vi "Window.vi"() -> ()   [LabVIEW 2010]
uses:
  <vilib>/Platform/TimedLoop/XDataNode/XDataNode.xnode
  <vilib>/Platform/TimedLoop/XDataNode/timing_clust.ctl
  <vilib>/Platform/TimedLoop/XDataNode/nitl_modes.ctl
  <vilib>/Platform/TimedLoop/XDataNode/wakeup.ctl
  LabView Dec.8/LabView Dec.8/SubVi's/Time Variable.vi
  SubVi's/Time Zone Offset.vi
  <vilib>/Utility/file.llb/Write To Spreadsheet File (string).vi
  LabView Dec.8/LabView Dec.8/SubVi's/Plot Variable.vi
  <vilib>/Platform/TimedLoop/XDataNode/XDNodeRunTimeDep.lvlib
  <vilib>/gmath/NI_Gmath.lvlib
  <vilib>/Analysis/NI_AALPro.lvlib
  LabView Dec.8/LabView Dec.8/SQL project lib.lvlib
  <vilib>/addons/database/NI_Database_API.lvlib
panel:
  in  "Background":bool
  in  "Grab Since Start":bool
  in  "Start Time":timestamp format="%<%H:%M:%S\n%x>T"
  in  "End Time":timestamp format="%<%H:%M:%S\n%x>T"
  in  "Grab Interval":bool
  in  "Fit":bool
  in  "Log(Y)":bool
  in  "Log(X)":bool
  in  "Remove":bool[](array[boolean])
  in  "Scatter/Histogram":bool=TRUE
  in  "bins":i32=250
  in  "min":dbl format="%_3g"
  in  "max":dbl=10.0 format="%0.2f"
  out "Current Data":dbl[](array[numeric])
  in  "Plot Scale":string[](array[string])=["y", "y", "y", "y", "y", "y", "y", "y", "y", "y", "y", "y", "y", "y", "y", "y", "y", "y", "y", "y", "y", "y", "y", "y", "y", "y", "y", "y", "y", "y", "y", "y", "y", "y", "y", "y", "y", "y", "y", "y", "y", "y", "y", "y", "y", "y", "y", "y", "y", "y", "y", "y", "y", "y", "y", "y", "y", "y", "y", "y", "y", "y", "y", "y", "y", "y", "y", "y", "y", "y", "y", "y", "y", "y", "y", "y", "y", "y", "y", "y", "y", "y", "y", "y", "y", "y", "y", "y", "y", "y", "y", "y", "y", "y", "y", "y", "y", "y", "y", "y", "y"]
  in  "Clear":bool
  out "Data Channel Name":string[](array[string])
  out "Realtime?":bool
  in  "Autoscale All":bool
  in  "output cluster":T1
  in  "Show Comments":bool
  in  "VI Refnum":refnum<vi>
  in  "Select Path (dialog if empty) 2":path
  in  "Save Front Panel Image":bool
  in  "Select Path (dialog if empty)":path
  in  "Write Data to \nLocal File":bool
  in  "Points to Plot":i32=4000
  in  "Realtime?":bool
  in  "Sent Array":cluster{dbl[], dbl[]}[](graph)
  in  "New String":string[](array[string])
  out "Plot":cluster{dbl[], dbl[]}[](graph)
  in  "New Data?":dbl=0.1
  out "Scaled Plot":cluster{dbl[], dbl[]}[](graph)
  # "Hist. Controls:"
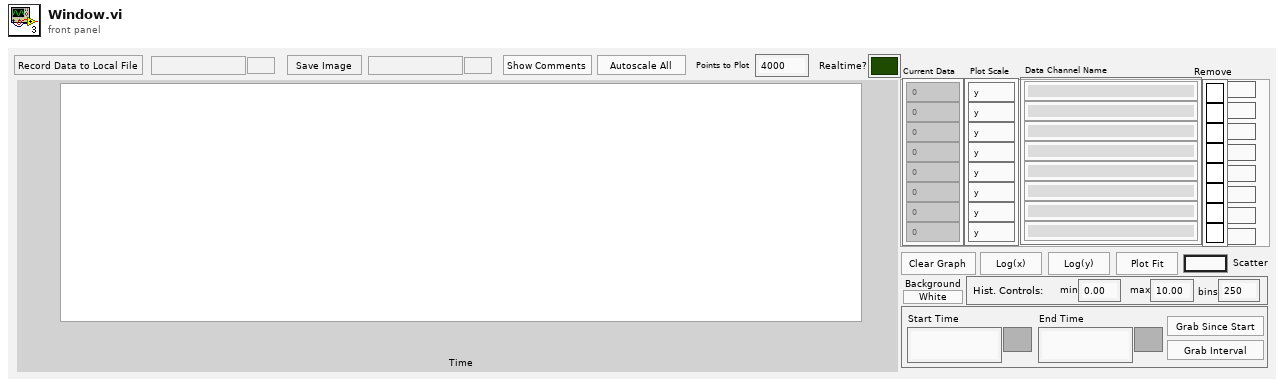
[diagram p1: front panel]
types:
  T1 = cluster{"Name":string, "Color":u32, "Style":u8, "Point Style":u8, "Name Visible":bool, "Allow Drag":bool, "Annotation Mode":u32, "Plot":i32, "Index":i32, "Position":cluster{"X":dbl, "Y":dbl}, "X Scale":u32, "Y Scale":u32, "Show Arrow":bool, "Lock Name":bool, "Plot Area":i32, "Label Offset":cluster{"X":dbl, "Y":dbl}}
  T2 = typedef "XDNodeRunTimeDep.lvlib/timing_clust.ctl" = cluster{"Expected End [f-1]":u64, "Actual End [f-1]":u64, "Finished Late? [f-1]":bool, "Expected End [i-1]":u64, "Actual End [i-1]":u64, "Finished Late? [i-1]":bool, "Expected Start [i]":u64, "Actual Start [i]":u64, "Expected Start [f]":u64, "Actual Start [f]":u64, "Source Name":string, "Structure Name":string, "Period":i64, "Deadline":i64, "Offset":i64, "Start":i64, "Priority":i32, "Timeout":i32, "Mode":T3, "Wakeup Reason":T4, "Error":errorcluster, "Source Type":string, "Secondary Source Type":string, "Global End Time":u64, "Global Start Time":u64, "Frame Duration":u64, "Iteration Duration":u64, "Assigned CPU":i32, "I/O Scan Engine Mode":u32}
  T3 = typedef "XDNodeRunTimeDep.lvlib/nitl_modes.ctl" = enum32{"No Change", "Process missed periods, maintain original phase", "Discard missed periods, maintain original phase", "Process missed periods, ignore original phase", "Discard missed periods, ignore original phase"}
  T4 = typedef "XDNodeRunTimeDep.lvlib/wakeup.ctl" = enum32{"Normal", "Aborted", "Asynchronous wakeup", "Timing source error", "Timed loop error", "Timeout"}
  T5 = typedef "LVAnnotationListTypeDef.ctl" = cluster{"Name":string, "Color":u32, "Style":u8, "Point Style":u8, "Name Visible":bool, "Allow Drag":bool, "Annotation Mode":u32, "Plot":i32, "Index":i32, "Position":cluster{"X":dbl, "Y":dbl}, "X Scale":u32, "Y Scale":u32, "Show Arrow":bool, "Lock Name":bool, "Plot Area":i32, "Label Offset":cluster{"X":dbl, "Y":dbl}}[]
  T6 = cluster{"X Values":dbl[], "Histogram: h(x)":i32[]}
  T7 = typedef "NI_Database_API.lvlib/Conn ObjectReference.ctl" = refnum<k1>
  T8 = typedef "imagedata.ctl" = cluster{"image type":i32, "image depth":i32, "image":u8[], "mask":u8[], "colors":u32[], "Rectangle":cluster{"left":i16, "top":i16, "right":i16, "bottom":i16}}
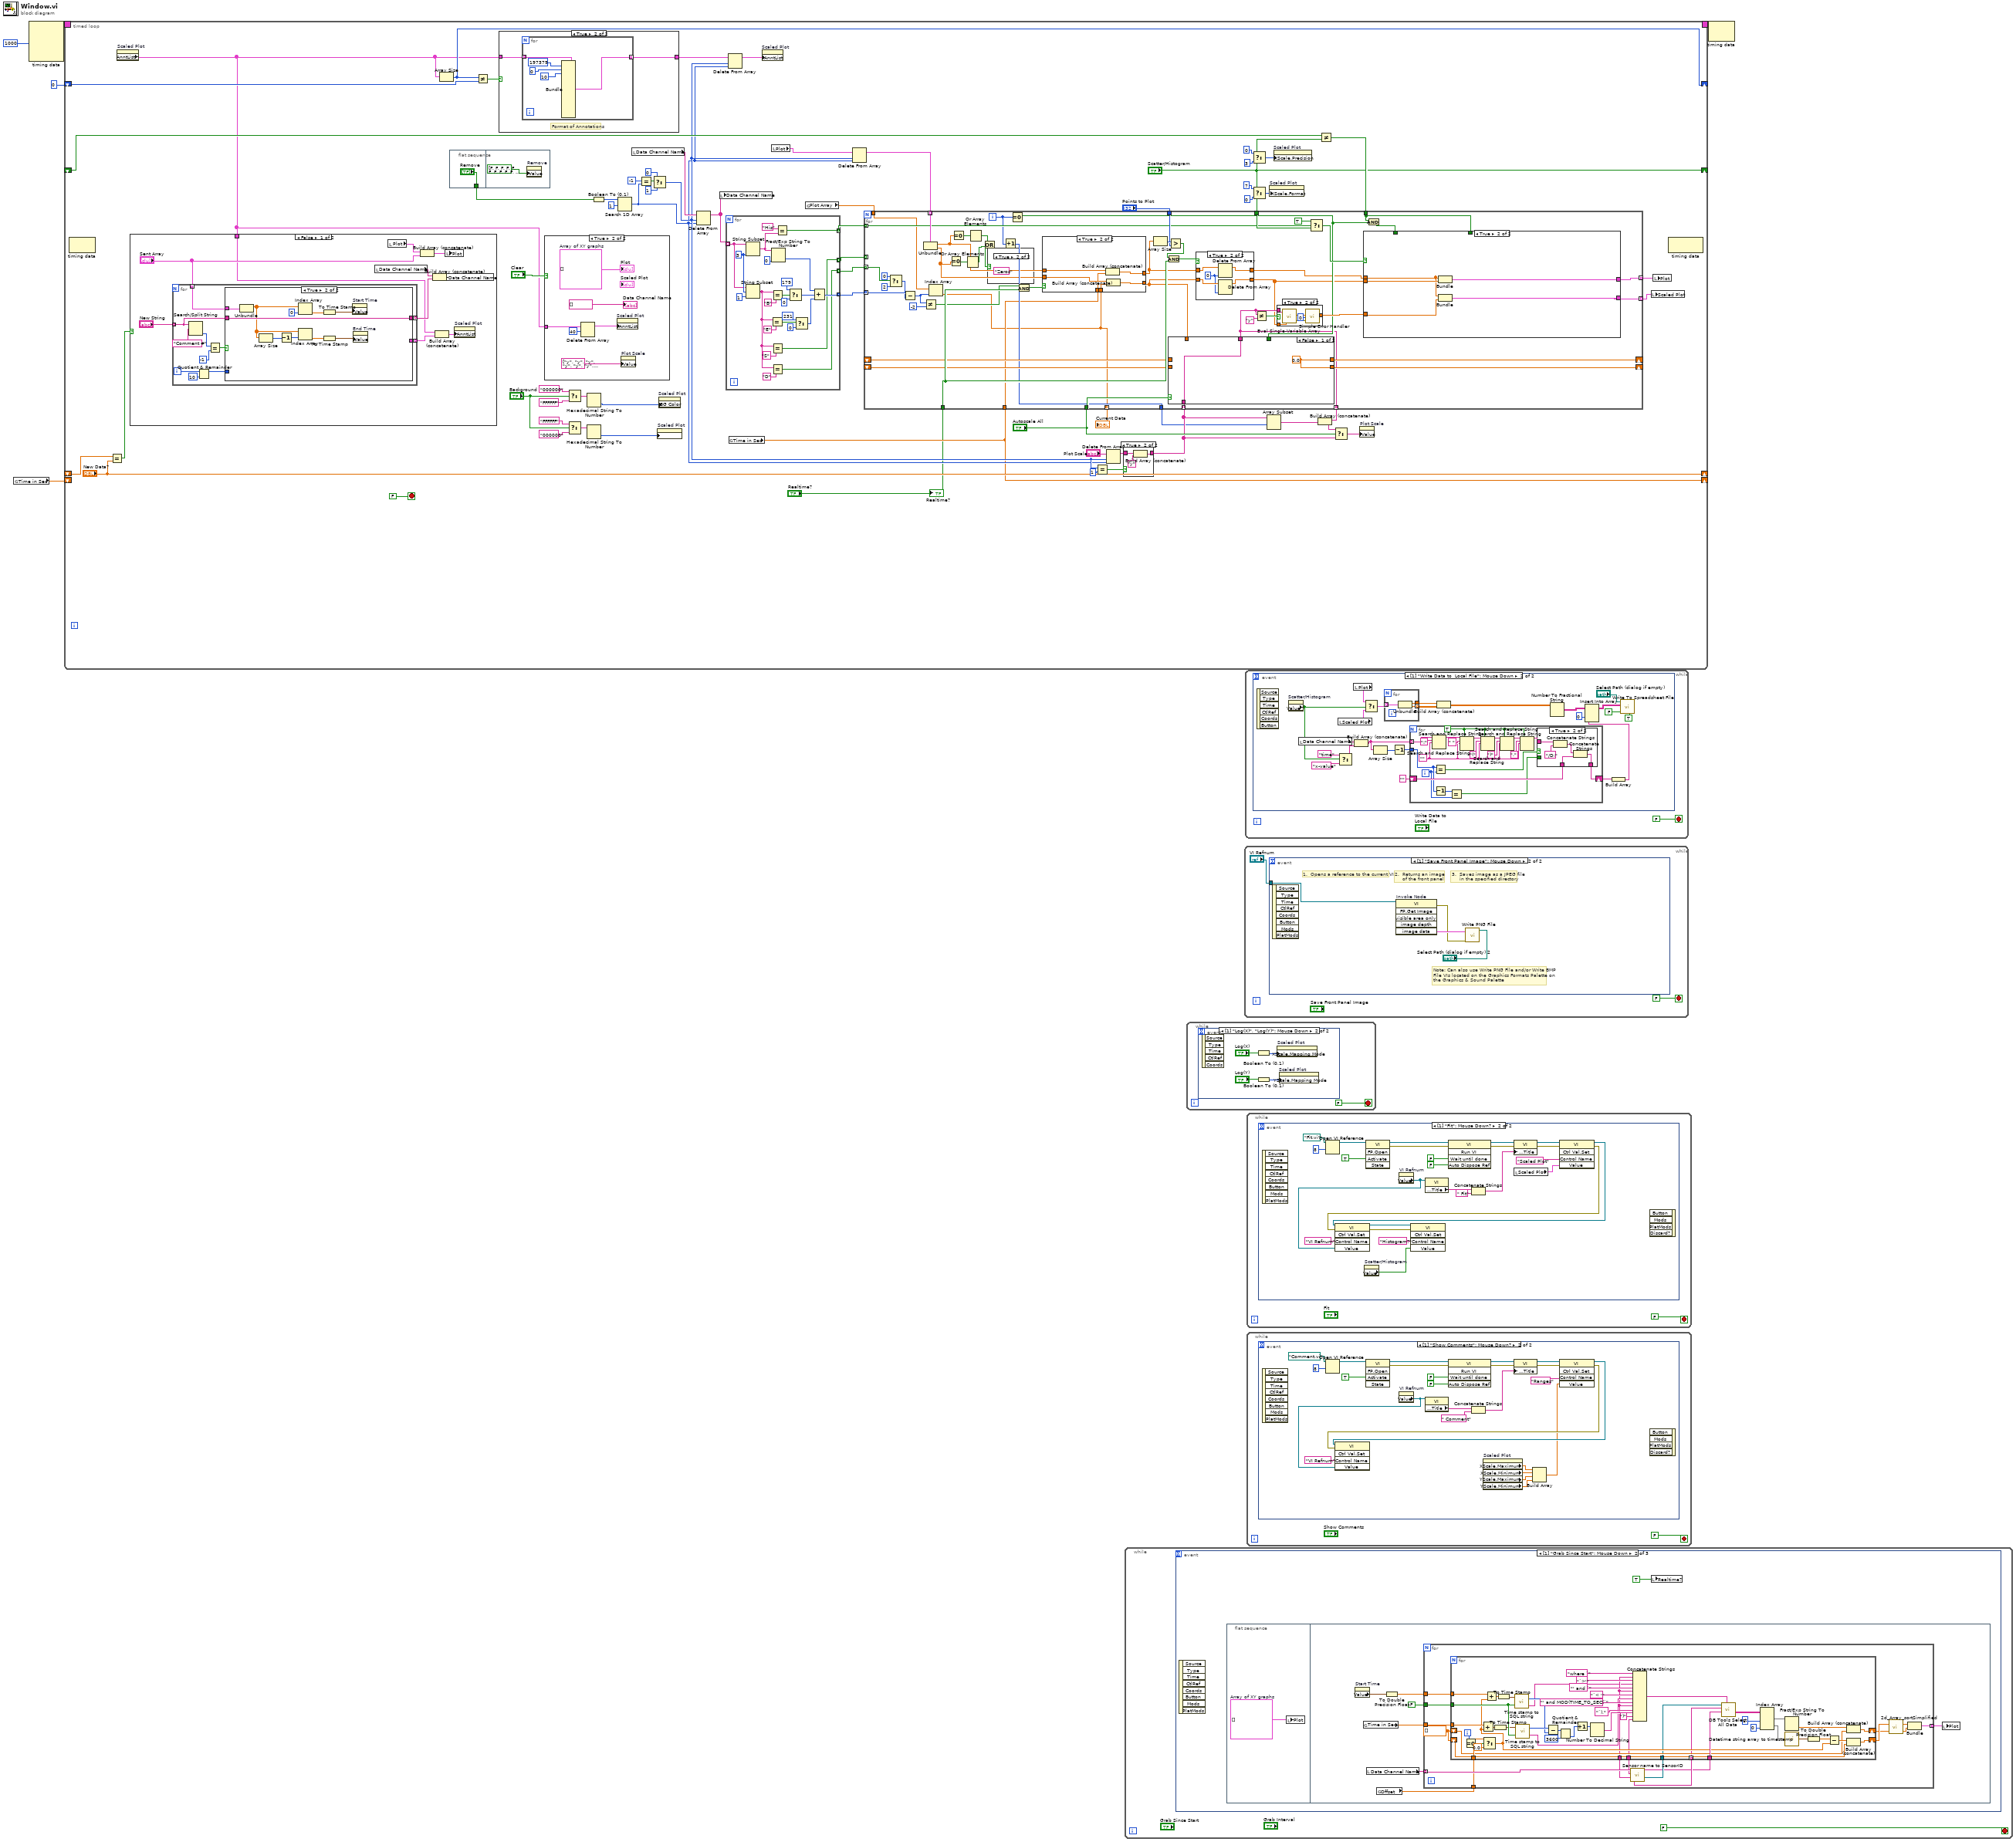
[diagram p0: block diagram]
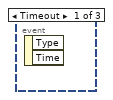
[diagram p2: hidden frame]
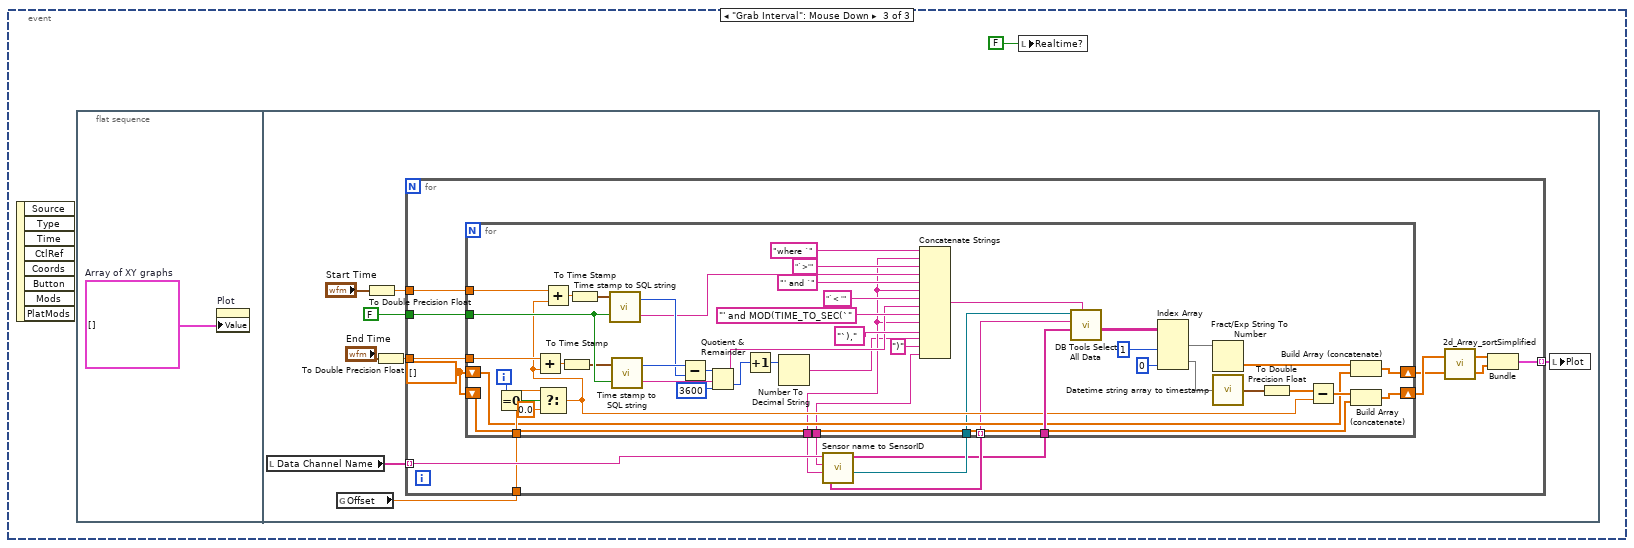
[diagram p3: hidden frame]
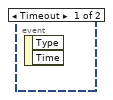
[diagram p4: hidden frame]
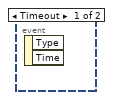
[diagram p5: hidden frame]
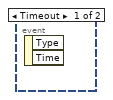
[diagram p6: hidden frame]
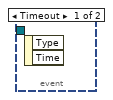
[diagram p7: hidden frame]
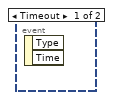
[diagram p8: hidden frame]
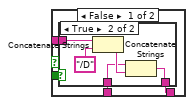
[diagram p9: hidden frame]
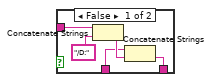
[diagram p10: hidden frame]
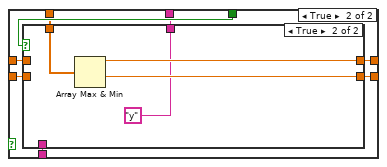
[diagram p15: hidden frame]
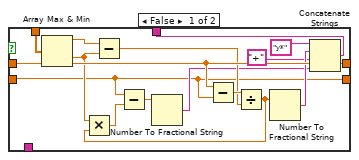
[diagram p16: hidden frame]
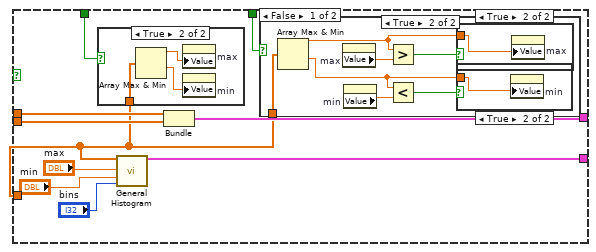
[diagram p18: hidden frame]
diagram:
  n1 = global read "Time Variable.vi" "Time in Sec"() -> (w1:dbl)
  n2 = node-c288(i64 1000 ("Period")) -> (w5:T2)  [unwired: 3 out]
  n3 = timed-loop {
    shift-right: ["New Data?"] -> _
    shift-left: _ -> [w67]
    timing: w5 -> [_]
    timing-out: [_] -> w4
    shift-right: ["Scatter/Histogram"] -> _
    shift-left: _ -> [w49]
    shift-right: [w46] -> _
    shift-left: 0 ("size(s)") -> [w47]
    shift-right: [w27] -> _
    shift-left: w1 -> [_]
    stop <- FALSE stop-if-true
    n4 = node-c288() -> ()  [unwired: 2 out]
    n5 = Equal?(x=w67, y="New Data?") -> (x = y?=w66:bool)
    n6 = property on="Scaled Plot" class="XYGraph (strict)"() -> ("AnntList"=w31:T5)  [unwired: 2 in, 2 out]
    n7 = case shown="False" w66 {
      tunnel: w31 -> [w245 _]
      frame False {
        n8 = for {
          tunnel: "New String" -> [w259] mode=indexing
          tunnel: "Sent Array" -> [w260] mode=indexing
          tunnel: [w258] -> w246 mode=indexing
          tunnel: [w257] -> w244 mode=indexing
          i -> [w256]
          n9 = Search/Split String(string=w259, search string/char (-)="Comment #") -> (offset of match=w262:i32)  [unwired: 3 out]
          n10 = Quotient & Remainder(x=w256, y=10) -> (x-y*floor(x/y)=w254:i32)  [unwired: 1 out]
          n11 = Equal?(x=w262, y=-1) -> (x = y?=w253:bool)
          n12 = case shown="True" w253 {
            tunnel: w260 -> [w283 w297]
            tunnel: w259 -> [w287 w298]
            tunnel: [w287 w298] -> w258
            tunnel: [w286 _] -> w257
            tunnel: w254 -> [w275 _]
            frame False {
              n13 = Unbundle(w283) -> (w282:dbl[], w279:dbl[])
              n14 = String Subset(string=w287, offset (0)=9) -> (substring=w285:string)  [unwired: 1 out]
              n15 = Index Array(array=w279, index #1=0 ("index"), index #2=1 ("index")) -> (element #1=w273:dbl, element #2=w266:dbl)
              n16 = Index Array(array=w282, index=0) -> (element=w264:dbl)
              n17 = Subtract(x=w273, y=w266) -> (x-y=w277:dbl)
              n18 = Divide(x=w277, y=12.0) -> (x/y=w272:dbl)
              n19 = Multiply(x=w272, y=w275) -> (x*y=w274:dbl)
              n20 = Compound Arithmetic op=ADD(w266, w272, w274) -> (w271:dbl)
              n21 = Bundle(w264, w271) -> (w284:cluster{dbl, dbl})  [unwired: 1 out]
              n22 = Bundle(cluster="output cluster", "Name"=w285, "Color"=u32 197379, "Style"=u8 0, "Point Style"=u8 10, "Name Visible"=TRUE, "Position"=w284) -> (w286:T1)  [unwired: 10 out]
            }
            frame True {
              n23 = Unbundle(w297) -> (w294:dbl[])  [unwired: 1 out]
              n24 = Array Size(array=w294) -> (size(s)=w295:i32)
              n25 = Decrement(x=w295) -> (x-1=w293:i32)
              n26 = Index Array(array=w294, index=w293) -> (element=w291:dbl)
              n27 = Index Array(array=w294, index=0) -> (element=w292:dbl)
              n28 = To Time Stamp(1:w292) -> (0:w290:timestamp)
              n29 = To Time Stamp(1:w291) -> (0:w289:timestamp)
              n30 = property on="Start Time" class="AbsTime (strict)"("Value"=w290) -> ()  [unwired: 2 in, 2 out]
              n31 = property on="End Time" class="AbsTime (strict)"("Value"=w289) -> ()  [unwired: 2 in, 2 out]
            }
          }
        }
        n32 = local read "Data Channel Name"() -> (w250:string[])
        n33 = local read "Plot"() -> (w251:cluster{dbl[], dbl[]}[])
        n34 = Build Array (concatenate)(w251, "Sent Array") -> (w252:cluster{dbl[], dbl[]}[])
        n35 = Build Array (concatenate)(w250, w246) -> (w249:string[])
        n36 = Build Array (concatenate)(w245, w244) -> (w243:T5)
        n37 = local write "Data Channel Name"(w249) -> ()
        n38 = local write "Plot"(w252) -> ()
        n39 = property on="Scaled Plot" class="XYGraph (strict)"("AnntList"=w243) -> ()  [unwired: 2 in, 2 out]
      }
      frame True {
      }
    }
    n40 = Array Size(array=w31) -> (size(s)=w46:i32)
    n41 = flat-sequence {
      tunnel: ["Remove"] -> w51
      frame #0 {
      }
      frame #1 {
        n42 = property on="Remove" class="Arr"("Value"=bool[] [FALSE, FALSE, FALSE, FALSE, FALSE, FALSE, FALSE, FALSE, FALSE, FALSE, FALSE, FALSE, FALSE, FALSE, FALSE, FALSE, FALSE, FALSE, FALSE, FALSE, FALSE] ("Array")) -> ()  [unwired: 2 in, 2 out]
      }
    }
    n43 = Not Equal?(x=w46, y=w47) -> (x != y?=w48:bool)
    n44 = case shown="True" w48 {
      tunnel: w31 -> [w98 w100]
      tunnel: [w98 w99] -> w35
      frame False {
      }
      frame True {
        # "Format of Annotations"
        n45 = for {
          tunnel: w100 -> [w105] mode=indexing
          tunnel: [w103] -> w99 mode=indexing
          n46 = Bundle(cluster=w105, "Color"=u32 197379, "Style"=u8 0, "Point Style"=u8 10) -> (w103:T1)  [unwired: 13 out]
        }
      }
    }
    n47 = case shown="True" "Clear" {
      tunnel: w31 -> [_ w240]
      frame False {
      }
      frame True {
        w241 = cluster{"Time":dbl[], "Y-values":dbl[]}[] []  # Array of XY graphs
        n48 = Delete From Array(array=w240, length=40) -> (array with subset deleted=w239:T5)  [unwired: 1 in, 1 out]
        n49 = property on="Scaled Plot" class="XYGraph (strict)"("AnntList"=w239) -> ()  [unwired: 2 in, 2 out]
        n50 = property on="Plot Scale" class="Arr (strict)"("Value"=string[] ["y", "y", "y", "y", "y", "y", "y", "y", "y", "y", "y", "y", "y", "y", "y", "y", "y", "y", "y", "y", "y", "y", "y", "y", "y", "y", "y", "y", "y", "y", "y", "y", "y", "y", "y", "y", "y", "y", "y", "y", "y", "y", "y", "y", "y", "y", "y", "y", "y", "y", "y", "y", "y", "y", "y", "y", "y", "y", "y", "y", "y", "y", "y", "y", "y", "y", "y", "y", "y", "y", "y", "y", "y", "y", "y", "y", "y", "y", "y", "y", "y", "y", "y", "y", "y", "y", "y", "y", "y", "y", "y", "y", "y", "y", "y", "y", "y", "y", "y", "y", "y"] ("Plot Scale 2")) -> ()  [unwired: 2 in, 2 out]
        "Plot" <- w241
        "Data Channel Name" <- string[] []
      }
    }
    n51 = Select(t="000000", s="Background", f="FFFFFF") -> (s? t:f=w17:string)
    n52 = Select(t="FFFFFF", s="Background", f="000000") -> (s? t:f=w10:string)
    n53 = Hexadecimal String To Number(string=w17) -> (number=w11:u32)  [unwired: 3 out]
    n54 = Hexadecimal String To Number(string=w10) -> (number=w9:u32)  [unwired: 3 out]
    n55 = Boolean To (0,1)(Boolean=w51) -> (0, 1=w58:i16[])
    n56 = Search 1D Array(1D array=w58, element=i16 1) -> (index of element=w32:i32)  [unwired: 1 out]
    n57 = local read "Data Channel Name"() -> (w59:string[])
    n58 = Equal?(x=-1 ("y"), y=w32) -> (x = y?=w56:bool)
    n59 = Select(t=0, s=w56, f=1 ("length")) -> (s? t:f=w33:i32)
    n60 = property on="Scaled Plot" class="XYGraph (strict)"("Plot.Plot Color"=w9) -> ()  [unwired: 2 in, 2 out]
    n61 = property on="Scaled Plot" class="XYGraph (strict)"("BG Color"=w11) -> ()  [unwired: 2 in, 2 out]
    n62 = Delete From Array(array=w59, length=w33, index=w32) -> (array with subset deleted=w30:string[])  [unwired: 1 out]
    n63 = local write "Data Channel Name"(w30) -> ()
    n64 = for {
      tunnel: w30 -> [w77] mode=indexing
      tunnel: [w76] -> w28 mode=indexing
      tunnel: [w75] -> w29 mode=indexing
      tunnel: [w73] -> w8 mode=indexing
      tunnel: [w70] -> w7 mode=indexing
      w92 = 3 ("length (rest)")
      n65 = String Subset(string=w77, length (rest)=w92) -> (substring=w79:string)  [unwired: 1 out]
      n66 = String Subset(string=w77, offset (0)=w92, length (rest)=1 ("length (rest)")) -> (substring=w71:string)
      n67 = Equal?(x=w71, y="E") -> (x = y?=w82:bool)
      n68 = Equal?(x=w71, y="B") -> (x = y?=w81:bool)
      n69 = Equal?(x=w71, y="S") -> (x = y?=w73:bool)
      n70 = Equal?(x=w71, y="D") -> (x = y?=w70:bool)
      n71 = Fract/Exp String To Number(string=w79, default (0 dbl)=0) -> (number=w84:i32)  [unwired: 3 out]
      n72 = Equal?(x="His", y=w79) -> (x = y?=w75:bool)
      n73 = Select(t=179, s=w81, f=0) -> (s? t:f=w88:i32)
      n74 = Select(t=231, s=w82, f=0) -> (s? t:f=w80:i32)
      n75 = Compound Arithmetic op=ADD(w84, w88, w80) -> (w76:i32)
    }
    n76 = Delete From Array(array=w35, length=w33, index=w32) -> (array with subset deleted=w34:T5)  [unwired: 1 out]
    n77 = global read "Time Variable.vi" "Time in Sec"() -> (w27:dbl)
    n78 = property on="Scaled Plot" class="XYGraph (strict)"("AnntList"=w34) -> ()  [unwired: 2 in, 2 out]
    n79 = local read "Plot"() -> (w6:cluster{dbl[], dbl[]}[])
    n80 = global read "Plot Variable.vi" "Plot Array"() -> (w60:dbl[])
    n81 = Delete From Array(array=w6, length=w33, index=w32) -> (array with subset deleted=w26:cluster{dbl[], dbl[]}[])  [unwired: 1 out]
    n82 = Equal?(x=w33, y=1) -> (x = y?=w44:bool)
    n83 = Delete From Array(array="Plot Scale", length=w33, index=w32) -> (array with subset deleted=w45:string[])  [unwired: 1 out]
    n84 = case shown="True" w44 {
      tunnel: w45 -> [w94 w97]
      tunnel: [w94 w96] -> w19
      frame False {
      }
      frame True {
        n85 = Build Array (concatenate)(w97, "y" ("x")) -> (w96:string[])
      }
    }
    n86 = Select(t=u8 0 ("X Scale.Display Format:Format"), s="Scatter/Histogram", f=u8 3) -> (s? t:f=w37:u8)
    n87 = Select(t=u8 7 ("X Scale.Display Format:Format"), s="Scatter/Histogram", f=u8 0) -> (s? t:f=w42:u8)
    n88 = property on="Scaled Plot" class="XYGraph (strict)"("XScale.Format"=w42) -> ()  [unwired: 2 in, 2 out]
    n89 = property on="Scaled Plot" class="XYGraph (strict)"("XScale.Precision"=w37) -> ()  [unwired: 2 in, 2 out]
    n90 = Not Equal?(x=w49, y="Scatter/Histogram") -> (x != y?=w50:bool)
    n91 = for {
      tunnel: w26 -> [w157] mode=indexing
      tunnel: w27 -> [w120]
      tunnel: w60 -> [w121]
      tunnel: [w156] -> w63 mode=indexing
      tunnel: "Points to Plot" -> [w154]
      tunnel: w19 -> [w134] mode=indexing
      tunnel: [w119] -> w62 mode=indexing
      tunnel: [w151] -> w61 mode=indexing
      tunnel: "Scatter/Histogram" -> [w143]
      tunnel: w50 -> [w146]
      tunnel: "Realtime?" -> [w137]
      tunnel: w28 -> [w142] mode=indexing
      tunnel: w29 -> [w141] mode=indexing
      tunnel: "Autoscale All" -> [w135]
      shift-right: [w132] -> _
      shift-left: _ -> [w130]
      shift-right: [w131] -> _
      shift-left: _ -> [w129]
      tunnel: [w128] -> w22 mode=indexing
      tunnel: [w126] -> w18
      tunnel: w8 -> [_] mode=indexing
      tunnel: w7 -> [w125] mode=indexing
      i -> [w127]
      n92 = Select(t=0, s=w125, f=2 ("y")) -> (s? t:f=w122:i32)
      n93 = Subtract(x=w142, y=w122) -> (x-y=w140:i32)
      n94 = Unbundle(w157) -> (w114:dbl[], w113:dbl[])
      n95 = Not Equal?(x=w140, y=-2) -> (x != y?=w136:bool)
      n96 = Index Array(array=w121, index=w140) -> (element=w119:dbl)
      n97 = Equal To 0?(x=w113) -> (x = 0?=w111:bool[])
      n98 = Equal To 0?(x=w114) -> (x = 0?=w112:bool[])
      n99 = Or Array Elements(Boolean array=w111) -> (logical OR=w109:bool)
      n100 = Or Array Elements(Boolean array=w112) -> (logical OR=w110:bool)
      n101 = Or(x=w110, y=w109) -> (x .or. y?=w108:bool)
      n102 = case shown="True" w108 {
        frame False {
        }
        frame True {
          (unwired) "Zeros"
        }
      }
      n103 = Increment(x=w127) -> (x+1=w126:i32)
      n104 = Equal To 0?(x=w127) -> (x = 0?=w133:bool)
      n105 = Compound Arithmetic op=AND(w136, w137) -> (w138:bool)
      n106 = case shown="True" w138 {
        tunnel: w113 -> [w158 w165]
        tunnel: w120 -> [_ w164]
        tunnel: w114 -> [w159 w163]
        tunnel: [w159 w162] -> w118
        tunnel: [w158 w161] -> w117
        tunnel: w119 -> [_ w160]
        frame False {
        }
        frame True {
          n107 = Build Array (concatenate)(w163, w164) -> (w162:dbl[])
          n108 = Build Array (concatenate)(w165, w160) -> (w161:dbl[])
        }
      }
      n109 = Array Size(array=w118) -> (size(s)=w155:i32)
      n110 = case shown="False" w135 {
        tunnel: w134 -> [w167 w168]
        tunnel: [w167 w169] -> w128
        tunnel: w133 -> [_ w175]
        tunnel: w117 -> [_ w174]
        tunnel: [w166 w173] -> w132
        tunnel: [w166 w172] -> w131
        tunnel: w130 -> [_ w171]
        tunnel: w129 -> [_ w170]
        frame False {
          w166 = 0.0
        }
        frame True {
          n111 = case shown="True" w175 {
            tunnel: w174 -> [w190 w194]
            tunnel: [w189 w193] -> w173
            tunnel: [w177 w192] -> w172
            tunnel: w171 -> [w189 _]
            tunnel: w170 -> [w177 _]
            tunnel: [w184 "y" ("x")] -> w169
            tunnel: w168 -> [_ _]
            frame False {
              n112 = Array Max & Min(array=w190) -> (max value=w187:dbl, min value=w178:dbl)  [unwired: 2 out]
              n113 = Subtract(x=w187, y=w178) -> (x-y=w186:dbl)
              n114 = Subtract(x=w189, y=w177) -> (x-y=w188:dbl)
              n115 = Divide(x=w188, y=w186) -> (x/y=w179:dbl)
              n116 = Multiply(x=w178, y=w179) -> (x*y=w180:dbl)
              n117 = Subtract(x=w177, y=w180) -> (x-y=w176:dbl)
              n118 = Number To Fractional String(number=w176) -> (F-format string=w181:string)  [unwired: 3 out]
              n119 = Number To Fractional String(number=w179) -> (F-format string=w183:string)  [unwired: 3 out]
              n120 = Concatenate Strings("y*" ("x"), w183, "+" ("x"), w181) -> (w184:string)
            }
            frame True {
              n121 = Array Max & Min(array=w194) -> (max value=w193:dbl, min value=w192:dbl)  [unwired: 2 out]
            }
          }
        }
      }
      n122 = Greater?(x=w155, y=w154) -> (0:w153:bool)
      n123 = And(x=w153, y=w137) -> (x .and. y?=w152:bool)
      n124 = case shown="True" w152 {
        tunnel: w118 -> [w229 w232]
        tunnel: w117 -> [w228 w233]
        tunnel: [w229 w234] -> w115
        tunnel: [w228 w231] -> w116
        frame False {
        }
        frame True {
          w230 = 0 ("length")
          n125 = Delete From Array(array=w232, index=w230) -> (array with subset deleted=w234:dbl[])  [unwired: 1 in, 1 out]
          n126 = Delete From Array(array=w233, index=w230) -> (array with subset deleted=w231:dbl[])  [unwired: 1 in, 1 out]
        }
      }
      n127 = Not Equal?(x=w128, y="y" ("x")) -> (x != y?=w150:bool)
      n128 = case shown="True" w150 {
        tunnel: w116 -> [w195 w200]
        tunnel: [w195 w199] -> w148
        tunnel: w128 -> [_ w198]
        frame False {
        }
        frame True {
          n129 = call <vilib>:"Eval Single-Variable Array.vi"("X Values"=w200, "formula"=w198) -> ("error out"=w196:errorcluster, "Y Values"=w199:dbl[])  [unwired: 1 in]
          n130 = call <vilib>:"Simple Error Handler.vi"("type of dialog (OK msg:1)"=i8 0 ("y"), "error in (no error)"=w196) -> ()  [unwired: 8 out]
        }
      }
      n131 = Select(t=TRUE, s=w141, f=w143) -> (s? t:f=w145:bool)
      n132 = And(x=w146, y=w133) -> (x .and. y?=w147:bool)
      n133 = case shown="True" w145 {
        tunnel: [w209 w227] -> w156
        tunnel: w116 -> [w207 w226]
        tunnel: w115 -> [w208 w225]
        tunnel: [w210 w224] -> w151
        tunnel: w148 -> [w201 w223]
        tunnel: w147 -> [w203 _]
        tunnel: w146 -> [w202 _]
        frame False {
          n134 = case shown="True" w203 {
            tunnel: w201 -> [_ w222]
            frame False {
            }
            frame True {
              n135 = Array Max & Min(array=w222) -> (max value=w221:dbl, min value=w220:dbl)  [unwired: 2 out]
              n136 = property on="max" class="DigNum (strict)"("Value"=w221) -> ()  [unwired: 2 in, 2 out]
              n137 = property on="min" class="DigNum (strict)"("Value"=w220) -> ()  [unwired: 2 in, 2 out]
            }
          }
          n138 = call <vilib>:"General Histogram.vi"("X"=w201, "max"="max", "min"="min", "# bins"="bins") -> ("Histogram Graph"=w210:T6)  [unwired: 2 in, 9 out]
          n139 = Bundle(w208, w207) -> (w209:cluster{dbl[], dbl[]})  [unwired: 1 out]
          n140 = case shown="True" w202 {
            tunnel: w201 -> [_ w217]
            frame False {
            }
            frame True {
              n141 = Array Max & Min(array=w217) -> (max value=w213:dbl, min value=w211:dbl)  [unwired: 2 out]
              n142 = property on="max" class="DigNum (strict)"() -> ("Value"=w216:dbl)  [unwired: 2 in, 2 out]
              n143 = property on="min" class="DigNum (strict)"() -> ("Value"=w215:dbl)  [unwired: 2 in, 2 out]
              n144 = Greater?(x=w213, y=w216) -> (0:w214:bool)
              n145 = Less?(x=w211, y=w215) -> (x < y?=w212:bool)
              n146 = case shown="True" w214 {
                tunnel: w213 -> [_ w219]
                frame False {
                }
                frame True {
                  n147 = property on="max" class="DigNum (strict)"("Value"=w219) -> ()  [unwired: 2 in, 2 out]
                }
              }
              n148 = case shown="True" w212 {
                tunnel: w211 -> [_ w218]
                frame False {
                }
                frame True {
                  n149 = property on="min" class="DigNum (strict)"("Value"=w218) -> ()  [unwired: 2 in, 2 out]
                }
              }
            }
          }
        }
        frame True {
          n150 = Bundle(w225, w226) -> (w227:cluster{dbl[], dbl[]})  [unwired: 1 out]
          n151 = Bundle(w225, "Y Values"=w223) -> (w224:cluster{dbl[], "Y Values":dbl[]})  [unwired: 1 out]
        }
      }
    }
    "Current Data" <- w62
    n152 = Array Subset(array=w19, index=w18) -> (w20:string[])  [unwired: 1 in]
    n153 = Build Array (concatenate)(w22, w20) -> (w21:string[])
    n154 = Select(t=w21, s="Autoscale All", f=w19) -> (s? t:f=w24:string[])
    n155 = property on="Plot Scale" class="Arr (strict)"("Value"=w24) -> ()  [unwired: 2 in, 2 out]
    n156 = local write "Scaled Plot"(w61) -> ()
    n157 = local write "Plot"(w63) -> ()
    n158 = node-c288() -> ()  [unwired: 2 out]
    "Realtime?" <- "Realtime?"
  }
  n159 = while {
    stop <- FALSE ("stop 2") stop-if-true
    n160 = event shown="[1] \"Grab Since Start\": Mouse Down" {
      selector: _ -> [_ _ _]
      dyn-events: _ -> [_ _ _]
      timeout: _ -> [_ _ _]
      event Timeout {
        n161 = event-data() -> ()  [unwired: 3 out]
      }
      event "Grab Since Start": Mouse Down {
        n162 = event-data() -> ()  [unwired: 9 out]
        n163 = flat-sequence {
          frame #0 {
            w301 = cluster{"Time":dbl[], "Y-values":dbl[]}[] []  # Array of XY graphs
            n164 = local write "Plot"(w301) -> ()
          }
          frame #1 {
            n165 = property on="Start Time" class="AbsTime (strict)"() -> ("Value"=w308:timestamp)  [unwired: 2 in, 2 out]
            n166 = global read "Time Variable.vi" "Time in Sec"() -> (w305:dbl)
            n167 = local read "Data Channel Name"() -> (w303:string[])
            n168 = global read "Time Zone Offset.vi" "Offset"() -> (w304:dbl)
            n169 = To Double Precision Float(number=w308) -> (double precision float=w307:dbl)
            n170 = for {
              tunnel: FALSE ("SQL formatting?") -> [w324]
              tunnel: w307 -> [w323]
              tunnel: w305 -> [w322]
              tunnel: w303 -> [w321] mode=indexing
              tunnel: [w320] -> w302 mode=indexing
              tunnel: w304 -> [w317]
              w314 = dbl[] []
              n171 = call "Sensor name to SensorID.vi"("Sensor name"=w321) -> ("Database Connection"=w312:T7, "Column Names"=w311:string[], "TableNameArray"=w313:string[], "Time Name"=w310:string, "Modulus Number"=w309:string)  [unwired: 2 out]
              n172 = for {
                tunnel: w324 -> [w371]
                tunnel: w323 -> [w370]
                tunnel: w322 -> [w369]
                tunnel: w311 -> [w363]
                tunnel: w317 -> [w347]
                shift-right: [w344] -> w315
                shift-left: w314 -> [w340]
                shift-right: [w342] -> w316
                shift-left: w314 -> [w341]
                tunnel: w313 -> [w339] mode=indexing
                tunnel: w312 -> [w338]
                tunnel: w310 -> [w326]
                tunnel: w309 -> [w330]
                i -> [w349]
                n173 = Equal To 0?(x=w349) -> (x = 0?=w351:bool)
                n174 = Select(t=w347, s=w351, f=0.0) -> (s? t:f=w346:dbl)
                n175 = Add(x=w369, y=w346) -> (x+y=w353:dbl)
                n176 = Add(x=w370, y=w346) -> (x+y=w355:dbl)
                n177 = To Time Stamp(1:w353) -> (0:w352:timestamp)
                n178 = To Time Stamp(1:w355) -> (0:w354:timestamp)
                n179 = call "Time stamp to SQL string.vi"("SQL formatting?"=w371, "time stamp"=w354) -> ("SQL format date-time string"=w325:string, "Seconds Since 1904"=w360:i64)
                n180 = call "Time stamp to SQL string.vi"("SQL formatting?"=w371, "time stamp"=w352) -> ("SQL format date-time string"=w327:string, "Seconds Since 1904"=w361:i64)
                n181 = Subtract(x=w361, y=w360) -> (x-y=w359:i64)
                n182 = Quotient & Remainder(x=w359, y=i64 3600) -> (floor(x/y)=w357:i64)  [unwired: 1 out]
                n183 = Increment(x=w357) -> (x+1=w356:i64)
                n184 = Number To Decimal String(number=w356) -> (decimal integer string=w328:string)  [unwired: 1 out]
                n185 = Concatenate Strings("where `" ("optional clause"), w326, "`>'" ("optional clause"), w325, "' and `" ("optional clause"), w326, "`< '" ("optional clause"), w327, "' and MOD(TIME_TO_SEC(`" ("optional clause"), w326, "`)," ("optional clause"), w328, ")" ("optional clause"), w330) -> (w331:string)
                n186 = call <vilib>:"DB Tools Select All Data.vi"("optional clause"=w331, "columns"=w363, "table"=w339, "connection reference"=w338) -> ("data"=w348:string[][])  [unwired: 1 in, 3 out]
                n187 = Index Array(array=w348, index (col) #1=1 ("disabled index (col)"), index (col) #2=0 ("index (col)")) -> (element #1=w367:string[], element #2=w365:string[])  [unwired: 2 in]
                n188 = Fract/Exp String To Number(string=w367) -> (number=w345:dbl[])  [unwired: 4 out]
                n189 = call "Datetime string array to timestamp.vi"("Datetime string array"=w365) -> ("Time stamp array"=w364:timestamp[])
                n190 = To Double Precision Float(number=w364) -> (double precision float=w362:dbl[])
                n191 = Subtract(x=w362, y=w346) -> (x-y=w343:dbl[])
                n192 = Build Array (concatenate)(w345, w340) -> (w344:dbl[])
                n193 = Build Array (concatenate)(w343, w341) -> (w342:dbl[])
              }
              n194 = call "2d_Array_sortSimplified.vi"("Value"=w315, "Time"=w316) -> ("Dataout"=w318:dbl[], "Timeout"=w319:dbl[])
              n195 = Bundle("Timeout"=w319, "Dataout"=w318) -> (w320:cluster{"Timeout":dbl[], "Dataout":dbl[]})  [unwired: 1 out]
            }
            n196 = local write "Plot"(w302) -> ()
          }
        }
        n197 = local write "Realtime?"(TRUE ("stop 2")) -> ()
      }
      event "Grab Interval": Mouse Down {
        n198 = event-data() -> ()  [unwired: 9 out]
        n199 = flat-sequence {
          frame #0 {
            w373 = cluster{"Time":dbl[], "Y-values":dbl[]}[] []  # Array of XY graphs
            n200 = property on="Plot" class="XYGraph (strict)"("Value"=w373) -> ()  [unwired: 2 in, 2 out]
          }
          frame #1 {
            n201 = local read "Data Channel Name"() -> (w376:string[])
            n202 = global read "Time Zone Offset.vi" "Offset"() -> (w374:dbl)
            n203 = To Double Precision Float(number="Start Time") -> (double precision float=w380:dbl)
            n204 = To Double Precision Float(number="End Time") -> (double precision float=w378:dbl)
            n205 = for {
              tunnel: FALSE ("SQL formatting?") -> [w397]
              tunnel: w380 -> [w396]
              tunnel: w378 -> [w395]
              tunnel: w376 -> [w394] mode=indexing
              tunnel: [w393] -> w375 mode=indexing
              tunnel: w374 -> [w390]
              w387 = dbl[] []
              n206 = call "Sensor name to SensorID.vi"("Sensor name"=w394) -> ("Database Connection"=w385:T7, "Column Names"=w384:string[], "TableNameArray"=w386:string[], "Time Name"=w382:string, "Modulus Number"=w383:string)  [unwired: 2 out]
              n207 = for {
                tunnel: w397 -> [w444]
                tunnel: w396 -> [w443]
                tunnel: w395 -> [w442]
                tunnel: w384 -> [w436]
                tunnel: w390 -> [w420]
                shift-right: [w417] -> w388
                shift-left: w387 -> [w413]
                shift-right: [w415] -> w389
                shift-left: w387 -> [w414]
                tunnel: w386 -> [w412] mode=indexing
                tunnel: w385 -> [w411]
                tunnel: w383 -> [w401]
                tunnel: w382 -> [w400]
                i -> [w422]
                n208 = Equal To 0?(x=w422) -> (x = 0?=w424:bool)
                n209 = Select(t=w420, s=w424, f=0.0) -> (s? t:f=w419:dbl)
                n210 = Add(x=w442, y=w419) -> (x+y=w426:dbl)
                n211 = Add(x=w443, y=w419) -> (x+y=w428:dbl)
                n212 = To Time Stamp(1:w426) -> (0:w425:timestamp)
                n213 = To Time Stamp(1:w428) -> (0:w427:timestamp)
                n214 = call "Time stamp to SQL string.vi"("SQL formatting?"=w444, "time stamp"=w427) -> ("SQL format date-time string"=w403:string, "Seconds Since 1904"=w433:i64)
                n215 = call "Time stamp to SQL string.vi"("SQL formatting?"=w444, "time stamp"=w425) -> ("SQL format date-time string"=w402:string, "Seconds Since 1904"=w434:i64)
                n216 = Subtract(x=w434, y=w433) -> (x-y=w432:i64)
                n217 = Quotient & Remainder(x=w432, y=i64 3600) -> (floor(x/y)=w430:i64)  [unwired: 1 out]
                n218 = Increment(x=w430) -> (x+1=w429:i64)
                n219 = Number To Decimal String(number=w429) -> (decimal integer string=w399:string)  [unwired: 1 out]
                n220 = Concatenate Strings("where `" ("optional clause"), w400, "`>'" ("optional clause"), w403, "' and `" ("optional clause"), w400, "`< '" ("optional clause"), w402, "' and MOD(TIME_TO_SEC(`" ("optional clause"), w400, "`)," ("optional clause"), w399, ")" ("optional clause"), w401) -> (w398:string)
                n221 = call <vilib>:"DB Tools Select All Data.vi"("optional clause"=w398, "columns"=w436, "table"=w412, "connection reference"=w411) -> ("data"=w421:string[][])  [unwired: 1 in, 3 out]
                n222 = Index Array(array=w421, index (col) #1=1 ("disabled index (col)"), index (col) #2=0 ("index (col)")) -> (element #1=w440:string[], element #2=w438:string[])  [unwired: 2 in]
                n223 = Fract/Exp String To Number(string=w440) -> (number=w418:dbl[])  [unwired: 4 out]
                n224 = call "Datetime string array to timestamp.vi"("Datetime string array"=w438) -> ("Time stamp array"=w437:timestamp[])
                n225 = To Double Precision Float(number=w437) -> (double precision float=w435:dbl[])
                n226 = Subtract(x=w435, y=w419) -> (x-y=w416:dbl[])
                n227 = Build Array (concatenate)(w418, w413) -> (w417:dbl[])
                n228 = Build Array (concatenate)(w416, w414) -> (w415:dbl[])
              }
              n229 = call "2d_Array_sortSimplified.vi"("Value"=w388, "Time"=w389) -> ("Dataout"=w391:dbl[], "Timeout"=w392:dbl[])
              n230 = Bundle("Timeout"=w392, "Dataout"=w391) -> (w393:cluster{"Timeout":dbl[], "Dataout":dbl[]})  [unwired: 1 out]
            }
            n231 = local write "Plot"(w375) -> ()
          }
        }
        n232 = local write "Realtime?"(FALSE ("stop 2")) -> ()
      }
    }
  }
  n233 = while {
    stop <- FALSE ("stop") stop-if-true
    n234 = event shown="[1] \"Log(X)\", \"Log(Y)\": Mouse Down" {
      selector: _ -> [_ _]
      dyn-events: _ -> [_ _]
      timeout: _ -> [_ _]
      event Timeout {
        n235 = event-data() -> ()  [unwired: 3 out]
      }
      event "Log(X)", "Log(Y)": Mouse Down {
        n236 = event-data() -> ()  [unwired: 6 out]
        n237 = Boolean To (0,1)(Boolean="Log(X)") -> (0, 1=w447:i16)
        n238 = Boolean To (0,1)(Boolean="Log(Y)") -> (0, 1=w446:i16)
        n239 = property on="Scaled Plot" class="XYGraph (strict)"("XScale.Mapping Mode"=w447) -> ()  [unwired: 2 in, 2 out]
        n240 = property on="Scaled Plot" class="XYGraph (strict)"("YScale.Mapping Mode"=w446) -> ()  [unwired: 2 in, 2 out]
      }
    }
  }
  n241 = while {
    stop <- FALSE ("stop") stop-if-true
    n242 = event shown="[1] \"Save Front Panel Image\": Mouse Down" {
      selector: _ -> [_ _]
      dyn-events: _ -> [_ _]
      timeout: _ -> [_ _]
      tunnel: "VI Refnum" -> [_ w452]
      event Timeout {
        n243 = event-data() -> ()  [unwired: 3 out]
      }
      event "Save Front Panel Image": Mouse Down {
        # "Note: Can also use Write PNG File and/or Write BMP \nFile VIs located on the Graphics Formats Palette on\nthe Graphics & Sound Palette"
        # "3.  Saves image as a JPEG file\n     in the specified directory"
        # "2.  Returns an image \n     of the front panel"
        # "1.  Opens a reference to the current VI"
        n244 = event-data() -> ()  [unwired: 9 out]
        n245 = invoke on="Invoke Node" class="VI" method="FP.Get Image"(reference=w452) -> (error out=w454:errorcluster, "image data"=w455:T8)  [unwired: 5 in, 4 out]
        n246 = call <vilib>:"Write PNG File.vi"("error in (no error)"=w454, "image data"=w455, "path to PNG file"="Select Path (dialog if empty) 2") -> ()  [unwired: 9 out]
      }
    }
  }
  n247 = while {
    stop <- FALSE ("stop") stop-if-true
    n248 = event shown="[1] \"Write Data to \nLocal File\": Mouse Down" {
      selector: _ -> [_ _]
      dyn-events: _ -> [_ _]
      timeout: _ -> [_ _]
      event Timeout {
        n249 = event-data() -> ()  [unwired: 3 out]
      }
      event "Write Data to \nLocal File": Mouse Down {
        n250 = event-data() -> ()  [unwired: 7 out]
        n251 = property on="Scatter/Histogram" class="Bool (strict)"() -> ("Value"=w465:bool)  [unwired: 2 in, 2 out]
        n252 = local read "Data Channel Name"() -> (w461:string[])
        n253 = local read "Scaled Plot"() -> (w472:cluster{dbl[], dbl[]}[])
        n254 = Select(t="time" ("new element/subarray"), s=w465, f="x-value" ("new element/subarray")) -> (s? t:f=w462:string)
        n255 = local read "Plot"() -> (w473:cluster{dbl[], dbl[]}[])
        n256 = Build Array (concatenate)(w461, w462) -> (w460:string[])
        n257 = Select(t=w473, s=w465, f=w472) -> (s? t:f=w474:cluster{dbl[], dbl[]}[])
        n258 = Array Size(array=w460) -> (size(s)=w467:i32)
        n259 = for {
          tunnel: w474 -> [w521] mode=indexing
          tunnel: [w520] -> w479 mode=indexing
          tunnel: [w519] -> w478
          n260 = Unbundle(w521) -> (w519:dbl[], w520:dbl[])
        }
        n261 = Decrement(x=w467) -> (x-1=w466:i32)
        n262 = for {
          tunnel: w460 -> [w482] mode=indexing
          tunnel: w466 -> [w487]
          shift-right: [w488] -> w459
          shift-left: "" -> [w489]
          i -> [w485]
          w480 = ""
          w495 = TRUE ("replace all? (F)")
          n263 = Search and Replace String(input string=w482, search string=":", replace string=w480) -> (result string=w481:string)  [unwired: 1 in, 7 out]
          n264 = Equal?(x=w487, y=w485) -> (x = y?=w490:bool)
          n265 = Decrement(x=w487) -> (x-1=w486:i32)
          n266 = Equal?(x=w486, y=w485) -> (x = y?=w484:bool)
          n267 = Search and Replace String(replace all?=w495, input string=w481, search string=" ", replace string=w480) -> (result string=w498:string)  [unwired: 1 in, 6 out]
          n268 = Search and Replace String(replace all?=w495, input string=w498, search string="(", replace string=w480) -> (result string=w497:string)  [unwired: 1 in, 6 out]
          n269 = Search and Replace String(replace all?=w495, input string=w497, search string=")", replace string=w480) -> (result string=w496:string)  [unwired: 1 in, 6 out]
          n270 = Search and Replace String(replace all?=w495, input string=w496, search string=".", replace string=w480) -> (result string=w491:string)  [unwired: 1 in, 6 out]
          n271 = case shown="True" w490 {
            tunnel: w491 -> [w503 w518]
            tunnel: w489 -> [w502 w515]
            tunnel: [w500 w514] -> w488
            tunnel: w484 -> [w501 _]
            frame False {
              n272 = case shown="True" w501 {
                tunnel: w503 -> [w508 w511]
                tunnel: w502 -> [w505 w510]
                tunnel: [w504 w509] -> w500
                frame False {
                  n273 = Concatenate Strings(w508, "/D:" ("string")) -> (w506:string)
                  n274 = Concatenate Strings(w505, w506) -> (w504:string)
                }
                frame True {
                  n275 = Concatenate Strings(w511, "/D" ("string")) -> (w512:string)
                  n276 = Concatenate Strings(w510, w512) -> (w509:string)
                }
              }
            }
            frame True {
              n277 = Concatenate Strings(w518, "/D:" ("string")) -> (w516:string)
              n278 = Concatenate Strings(w516, w515) -> (w514:string)
            }
          }
        }
        n279 = Build Array (concatenate)(w478, w479) -> (w471:dbl[][])
        n280 = Number To Fractional String(number=w471) -> (F-format string=w470:string[][])  [unwired: 3 out]
        n281 = Build Array(w459) -> (w458:string[])
        n282 = Insert Into Array(array=w470, index (col)=0 ("disabled index (col)"), new element=w458) -> (w469:string[][])  [unwired: 1 in]
        n283 = call-poly <vilib>:"Write To Spreadsheet File.vi"("transpose? (no:F)"=TRUE, "append to file? (new file:F)"=FALSE, "2D data"=w469, "file path (dialog if empty)"="Select Path (dialog if empty)") -> ()  [unwired: 2 in, 3 out]
      }
    }
  }
  n284 = while {
    stop <- FALSE ("stop 2") stop-if-true
    n285 = event shown="[1] \"Fit\": Mouse Down?" {
      selector: _ -> [_ _]
      dyn-events: _ -> [_ _]
      timeout: _ -> [_ _]
      event Timeout {
        n286 = event-data() -> ()  [unwired: 3 out]
      }
      event "Fit": Mouse Down? {
        n287 = event-data() -> ()  [unwired: 9 out]
        n288 = Open VI Reference(vi path=path "Fit.vi", options=8) -> (vi reference=w538:refnum<vi>)  [unwired: 1 in, 4 out]
        n289 = property on="Scatter/Histogram" class="Bool (strict)"() -> ("Value"=w523:bool)  [unwired: 2 in, 2 out]
        n290 = invoke class="VI" method="FP.Open"(reference=w538, "Activate"=TRUE ("Activate?")) -> (reference out=w539:refnum<vi>, error out=w540:errorcluster)  [unwired: 3 in, 3 out]
        n291 = property on="VI Refnum" class="VIRef (strict)"() -> ("Value"=w530:refnum<vi>)  [unwired: 2 in, 2 out]
        n292 = property class="VI"(reference=w530) -> ("Front Panel.Title"=w529:string)  [unwired: 1 in, 2 out]
        n293 = invoke class="VI" method="Run VI"(reference=w539, error in=w540, "Wait until done"=FALSE ("Wait Until Done"), "Auto Dispose Ref"=FALSE ("Auto Dispose Reference")) -> (reference out=w543:refnum<vi>, error out=w544:errorcluster)  [unwired: 1 in, 3 out]
        n294 = Concatenate Strings(w529, " Fit" ("string")) -> (w528:string)
        n295 = property class="VI"(reference=w543, error in=w544, "Front Panel.Title"=w528) -> (reference out=w546:refnum<vi>, error out=w547:errorcluster)
        n296 = local read "Scaled Plot"() -> (w534:cluster{dbl[], dbl[]}[])
        n297 = invoke class="VI" method="Ctrl Val.Set"(reference=w546, error in=w547, "Control Name"="Scaled Plot", "Value"=w534) -> (reference out=w533:refnum<vi>, error out=w532:errorcluster)  [unwired: 1 in, 3 out]
        n298 = invoke class="VI" method="Ctrl Val.Set"(reference=w533, error in=w532, "Control Name"="VI Refnum", "Value"=w530) -> (reference out=w526:refnum<vi>, error out=w525:errorcluster)  [unwired: 1 in, 3 out]
        n299 = invoke class="VI" method="Ctrl Val.Set"(reference=w526, error in=w525, "Control Name"="Histogram?", "Value"=w523) -> ()  [unwired: 1 in, 5 out]
        n300 = event-data() -> ()  [unwired: 1 in, 5 out]
      }
    }
  }
  n301 = while {
    stop <- FALSE ("stop 2") stop-if-true
    n302 = event shown="[1] \"Show Comments\": Mouse Down?" {
      selector: _ -> [_ _]
      dyn-events: _ -> [_ _]
      timeout: _ -> [_ _]
      event Timeout {
        n303 = event-data() -> ()  [unwired: 3 out]
      }
      event "Show Comments": Mouse Down? {
        n304 = event-data() -> ()  [unwired: 9 out]
        n305 = Open VI Reference(vi path=path "Comment.vi", options=8) -> (vi reference=w564:refnum<vi>)  [unwired: 1 in, 4 out]
        n306 = invoke class="VI" method="FP.Open"(reference=w564, "Activate"=TRUE ("Activate?")) -> (reference out=w565:refnum<vi>, error out=w566:errorcluster)  [unwired: 3 in, 3 out]
        n307 = property on="VI Refnum" class="VIRef (strict)"() -> ("Value"=w557:refnum<vi>)  [unwired: 2 in, 2 out]
        n308 = property class="VI"(reference=w557) -> ("Front Panel.Title"=w556:string)  [unwired: 1 in, 2 out]
        n309 = invoke class="VI" method="Run VI"(reference=w565, error in=w566, "Wait until done"=FALSE ("Wait Until Done"), "Auto Dispose Ref"=FALSE ("Auto Dispose Reference")) -> (reference out=w569:refnum<vi>, error out=w570:errorcluster)  [unwired: 1 in, 3 out]
        n310 = Concatenate Strings(w556, " Comment" ("string")) -> (w555:string)
        n311 = property on="Scaled Plot" class="XYGraph (strict)"() -> ("XScale.Maximum"=w553:dbl, "XScale.Minimum"=w552:dbl, "YScale.Maximum"=w551:dbl, "YScale.Minimum"=w550:dbl)  [unwired: 2 in, 2 out]
        n312 = property class="VI"(reference=w569, error in=w570, "Front Panel.Title"=w555) -> (reference out=w572:refnum<vi>, error out=w573:errorcluster)
        n313 = Build Array(w553, w552, w551, w550) -> (w549:dbl[])
        n314 = invoke class="VI" method="Ctrl Val.Set"(reference=w572, error in=w573, "Control Name"="Ranges", "Value"=w549) -> (reference out=w560:refnum<vi>, error out=w559:errorcluster)  [unwired: 1 in, 3 out]
        n315 = invoke class="VI" method="Ctrl Val.Set"(reference=w560, error in=w559, "Control Name"="VI Refnum", "Value"=w557) -> ()  [unwired: 1 in, 5 out]
        n316 = event-data() -> ()  [unwired: 1 in, 5 out]
      }
    }
  }
  n317 = node-c288(w4) -> ()  [unwired: 1 out]
